vi "4bitNumericDemo.vi"() -> ()   [LabVIEW 2017]
panel:
  out "Numeric":dbl
  out "Gauge":dbl(knob) scale=0.0..15.0
  in  "Boolean 4":bool
  in  "Boolean 3":bool
  in  "Boolean 2":bool
  in  "Boolean":bool
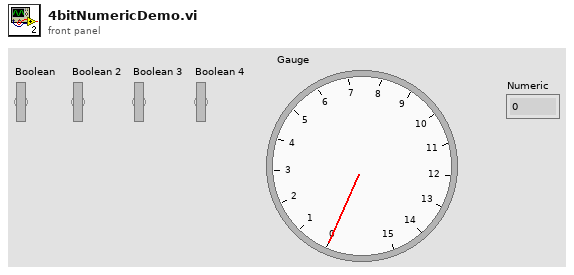
[diagram p1: front panel]
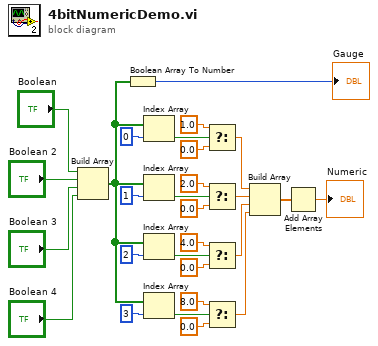
[diagram p0: block diagram]
diagram:
  n1 = Build Array("Boolean", "Boolean 2", "Boolean 3", "Boolean 4") -> (w7:bool[])
  n2 = Boolean Array To Number(Boolean array=w7) -> (number=→"Gauge":u32)
  n3 = Index Array(array=w7, index=0) -> (element=w20:bool)
  n4 = Index Array(array=w7, index=1) -> (element=w16:bool)
  n5 = Index Array(array=w7, index=2) -> (element=w12:bool)
  n6 = Index Array(array=w7, index=3) -> (element=w8:bool)
  n7 = Select(t=1.0, s=w20, f=0.0) -> (s? t:f=w6:dbl)
  n8 = Select(t=2.0, s=w16, f=0.0) -> (s? t:f=w5:dbl)
  n9 = Select(t=4.0, s=w12, f=0.0) -> (s? t:f=w4:dbl)
  n10 = Select(t=8.0, s=w8, f=0.0) -> (s? t:f=w3:dbl)
  n11 = Build Array(w6, w5, w4, w3) -> (w2:dbl[])
  n12 = Add Array Elements(numeric array=w2) -> (sum=→"Numeric":dbl)
